vi "DecodeTempAlert.vi"(11 "Message":string) -> (0 "High Limit":i16, 1 "Low Limit":i16, 3 "Temperature":dbl)   [LabVIEW 2012]
uses:
  TempMonitor_Command_Enumerations.vi
panel:
  out "High Limit String":string
  out "Low Limit String":string
  out "Temp String":string
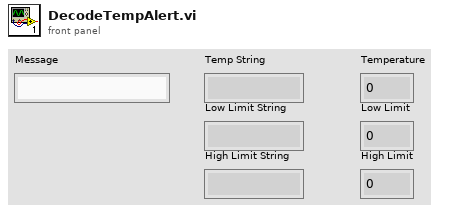
[diagram p1: front panel]
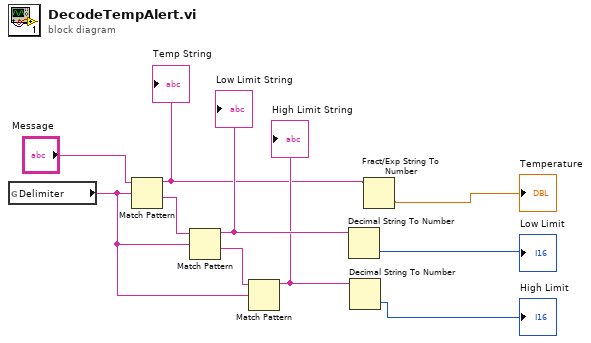
[diagram p0: block diagram]
diagram:
  n1 = global read "TempMonitor_Command_Enumerations.vi" "Delimiter"() -> (w7:string)
  n2 = Match Pattern(string="Message", regular expression=w7) -> (before substring=w4:string, after substring=w9:string)  [unwired: 1 in, 2 out]
  "Temp String" <- w4
  n3 = Match Pattern(string=w9, regular expression=w7) -> (before substring=w8:string, after substring=w6:string)  [unwired: 1 in, 2 out]
  "Low Limit String" <- w8
  n4 = Match Pattern(string=w6, regular expression=w7) -> (before substring=w5:string)  [unwired: 1 in, 3 out]
  "High Limit String" <- w5
  n5 = Decimal String To Number(string=w8) -> (number=→"Low Limit":i32)  [unwired: 2 in, 1 out]
  n6 = Decimal String To Number(string=w5) -> (number=→"High Limit":i32)  [unwired: 2 in, 1 out]
  n7 = Fract/Exp String To Number(string=w4) -> (number=→"Temperature":dbl)  [unwired: 3 in, 1 out]
